vi "Power Output Stimulus Key Array.vi"(4 "Conversion":enum16{"Cluster - HTML", "HTML - Cluster"}(ring), 6 "Stimulus Key Array In":T2, 7 "Stimulus Cluster In":T1) -> (1 "Stimulus Cluster Out":T1, 2 "Stimulus HTML Out":string)   [LabVIEW 2011]
uses:
  Addons/internet/utils/keyedarr.llb/Keyed Array.ctl
  TypeDefs/Power Output Stimulus Parameters.ctl
  Addons/internet/utils/strutil.llb/Case Matching.ctl
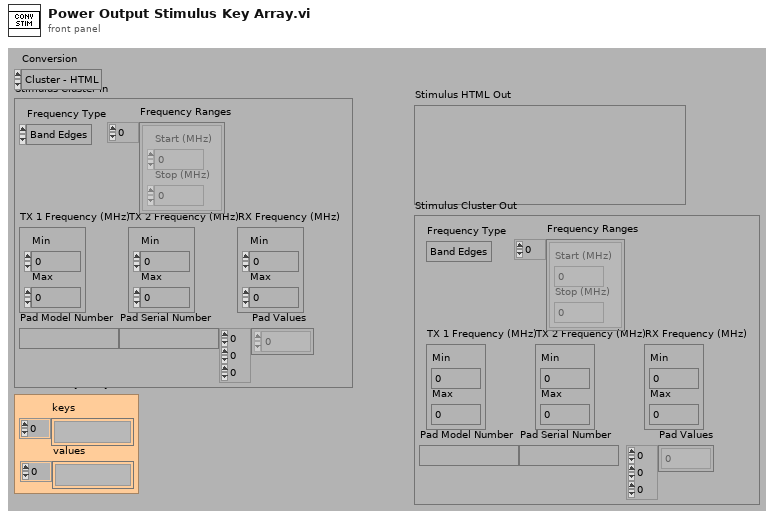
[diagram p1: front panel]
types:
  T1 = typedef "Power Output Stimulus Parameters.ctl" = cluster{"Frequency Type":enum16{"Band Edges", "Custom"}, "Frequency Ranges":cluster{"Start (MHz)":dbl, "Stop (MHz)":dbl}[], "TX 1 Frequency (MHz)":cluster{"Min":dbl, "Max":dbl}, "TX 2 Frequency (MHz)":cluster{"Min":dbl, "Max":dbl}, "RX Frequency (MHz)":cluster{"Min":dbl, "Max":dbl}, "Pad Model Number":string, "Pad Serial Number":string, "Pad Values":dbl[][][]}
  T2 = typedef "Keyed Array.ctl" = cluster{"keys":string[], "values":string[]}
  T3 = typedef "Case Matching.ctl" = enum16{"a != A", "a == A", "system"}
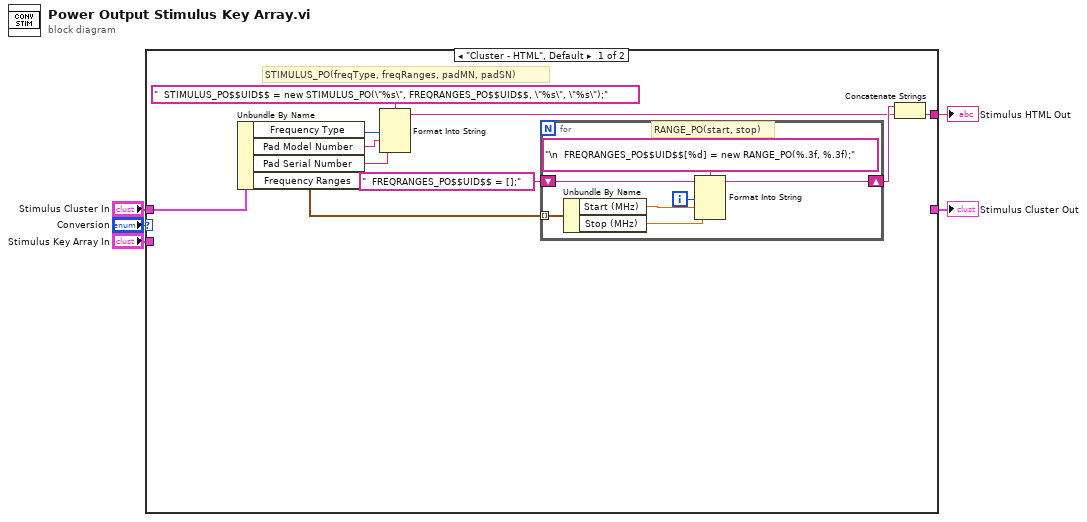
[diagram p0: block diagram]
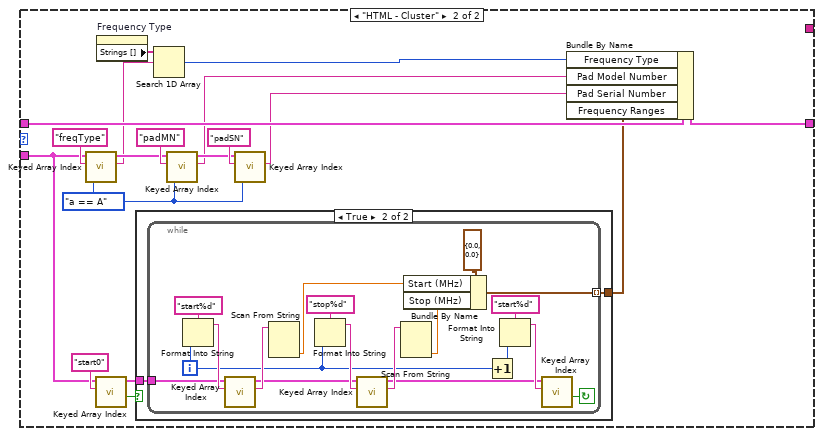
[diagram p2: hidden frame]
diagram:
  n1 = case shown="\"Cluster - HTML\", Default" "Conversion" {
    tunnel: "Stimulus Key Array In" -> [_ w26]
    tunnel: "Stimulus Cluster In" -> [w15 w40]
    tunnel: [w6 _] -> w3
    tunnel: [_ w39] -> w2
    frame "Cluster - HTML", Default {
      # "STIMULUS_PO(freqType, freqRanges, padMN, padSN)"
      n2 = Unbundle By Name(w15) -> ("Frequency Type"=w13:enum16{"Band Edges", "Custom"}, "Pad Model Number"=w11:string, "Pad Serial Number"=w12:string, "Frequency Ranges"=w9:cluster{"Start (MHz)":dbl, "Stop (MHz)":dbl}[])
      n3 = Format Into String(format string="  STIMULUS_PO$$UID$$ = new STIMULUS_PO(\"%s\", FREQRANGES_PO$$UID$$, \"%s\", \"%s\");", w13, w11, w12) -> (resulting string=w7:string)  [unwired: 2 in, 1 out]
      n4 = for {
        shift-right: [w20] -> w8
        shift-left: "  FREQRANGES_PO$$UID$$ = [];" ("format string") -> [w21]
        tunnel: w9 -> [w18] mode=indexing
        i -> [w19]
        # "RANGE_PO(start, stop)"
        n5 = Unbundle By Name(w18) -> ("Start (MHz)"=w17:dbl, "Stop (MHz)"=w16:dbl)
        n6 = Format Into String(format string="\n  FREQRANGES_PO$$UID$$[%d] = new RANGE_PO(%.3f, %.3f);", initial string=w21, w19, w17, w16) -> (resulting string=w20:string)  [unwired: 1 in, 1 out]
      }
      n7 = Concatenate Strings(w8, w7) -> (w6:string)
    }
    frame "HTML - Cluster" {
      w25 = Case_Matching."a == A" ("case matching (sensitive)")
      n8 = call "Keyed Array Index.vi"("case matching (sensitive)"=w25, "key"="freqType", "array in"=w26) -> ("value"=w23:string, "duplicate array"=w34:T2)  [unwired: 1 in, 2 out]
      n9 = call "Keyed Array Index.vi"("key"="start0", "array in"=w26) -> ("valid key"=w29:bool, "duplicate array"=w30:T2)  [unwired: 2 in, 2 out]
      n10 = property on="Frequency Type" class="Enum (strict)"() -> ("Strings []"=w24:string[])  [unwired: 2 in, 2 out]
      n11 = case shown="True" w29 {
        tunnel: w30 -> [_ w42]
        tunnel: [_ w41] -> w27
        frame False {
        }
        frame True {
          n12 = while {
            tunnel: w42 -> [w54]
            tunnel: [w43] -> w41 mode=indexing
            i -> [w47]
            stop <- w57 continue-if-true
            n13 = Format Into String(format string="start%d", w47) -> (resulting string=w55:string)  [unwired: 2 in, 1 out]
            n14 = call "Keyed Array Index.vi"("key"=w55, "array in"=w54) -> ("value"=w53:string, "duplicate array"=w49:T2)  [unwired: 2 in, 2 out]
            n15 = Scan From String(input string=w53) -> (output 1=w45:dbl)  [unwired: 4 in, 3 out]
            n16 = Format Into String(format string="stop%d", w47) -> (resulting string=w51:string)  [unwired: 2 in, 1 out]
            n17 = call "Keyed Array Index.vi"("key"=w51, "array in"=w49) -> ("value"=w52:string, "duplicate array"=w48:T2)  [unwired: 2 in, 2 out]
            n18 = Scan From String(input string=w52) -> (output 1=w44:dbl)  [unwired: 4 in, 3 out]
            n19 = Bundle By Name(cluster=cluster{"Start (MHz)":dbl, "Stop (MHz)":dbl} {"Start (MHz)"=0.0, "Stop (MHz)"=0.0}, "Start (MHz)"=w45, "Stop (MHz)"=w44) -> (w43:cluster{"Start (MHz)":dbl, "Stop (MHz)":dbl})
            n20 = Increment(x=w47) -> (x+1=w58:i32)
            n21 = Format Into String(format string="start%d", w58) -> (resulting string=w59:string)  [unwired: 2 in, 1 out]
            n22 = call "Keyed Array Index.vi"("key"=w59, "array in"=w48) -> ("valid key"=w57:bool)  [unwired: 2 in, 3 out]
          }
        }
      }
      n23 = Search 1D Array(1D array=w24, element=w23) -> (index of element=w31:i32)  [unwired: 1 out]
      n24 = call "Keyed Array Index.vi"("case matching (sensitive)"=w25, "key"="padMN", "array in"=w34) -> ("value"=w32:string, "duplicate array"=w37:T2)  [unwired: 1 in, 2 out]
      n25 = call "Keyed Array Index.vi"("case matching (sensitive)"=w25, "key"="padSN", "array in"=w37) -> ("value"=w33:string)  [unwired: 1 in, 3 out]
      n26 = Bundle By Name(cluster=w40, "Frequency Type"=w31, "Pad Model Number"=w32, "Pad Serial Number"=w33, "Frequency Ranges"=w27) -> (w39:T1)
    }
  }
  "Stimulus HTML Out" <- w3
  "Stimulus Cluster Out" <- w2
